vi "RSZVB Get Power Calibration Method Source.vi"(8 "error in (no error)":errorcluster {"code" format="%.0x"}, 11 "VISA resource name":refnum<visa-resource-name>) -> (0 "error out":errorcluster {"code" format="%.0x"}, 2 "Method Source":i32, 3 "VISA resource name out":refnum<visa-resource-name>)   [LabVIEW 2011]
doc: "This VI returns the source power calibration method. \n\nRemote-control command(s):\nSOURce<Ch>:POWer<Pt>:CORRection:COLLect:METHod?"
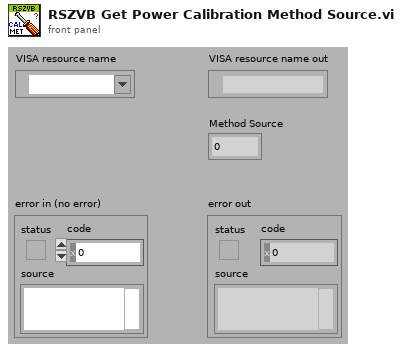
[diagram p1: front panel]
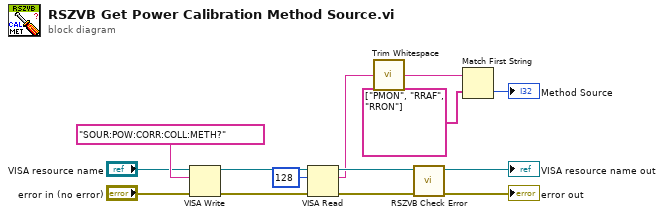
[diagram p0: block diagram]
diagram:
  n1 = VISA Write(VISA resource name="VISA resource name", write buffer="SOUR:POW:CORR:COLL:METH?" ("format string"), error in (no error)="error in (no error)") -> (VISA resource name out=w11:refnum<visa-resource-name>, error out=w10:errorcluster)  [unwired: 1 out]
  n2 = VISA Read(VISA resource name=w11, byte count=u32 128, error in (no error)=w10) -> (VISA resource name out=w8:refnum<visa-resource-name>, read buffer=w4:string, error out=w9:errorcluster)  [unwired: 1 out]
  n3 = call <vilib>:"Trim Whitespace.vi"("string"=w4) -> ("trimmed string"=w1:string)  [unwired: 1 in]
  n4 = call "RSZVB Check Error.vi"("error in (no error)"=w9, "VISA session"=w8) -> ("error out"=→"error out":errorcluster, "dup VISA session"=→"VISA resource name out":refnum<visa-resource-name>)  [unwired: 8 in]
  n5 = Match First String(2:string[] ["PMON", "RRAF", "RRON"], 3:w1) -> (0:→"Method Source":i32)  [unwired: 1 out]
